vi "PDExitByError.vi"(1 "ExitLimit":dbl, 2 "Time(s)":dbl, 3 "NewValue":dbl) -> (0 "ShouldExit?":bool)   [LabVIEW 2016]
uses:
  <vilib>/Analysis/NI_AALBase.lvlib
  <vilib>/Analysis/baseanly.llb/Mean (DBL).vi
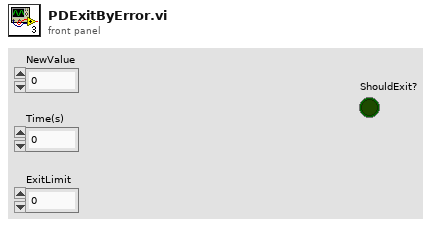
[diagram p1: front panel]
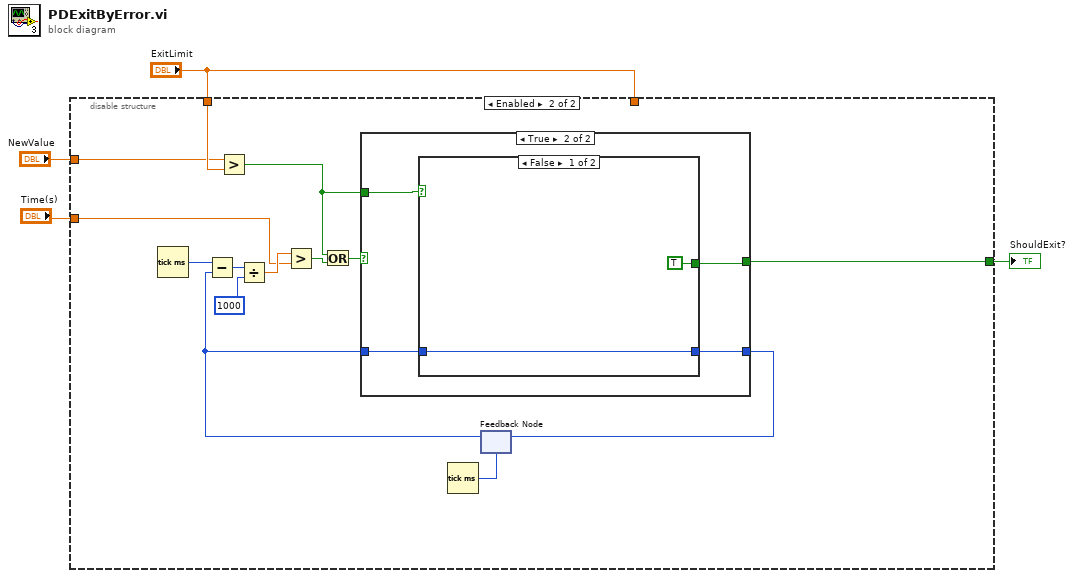
[diagram p0: block diagram]
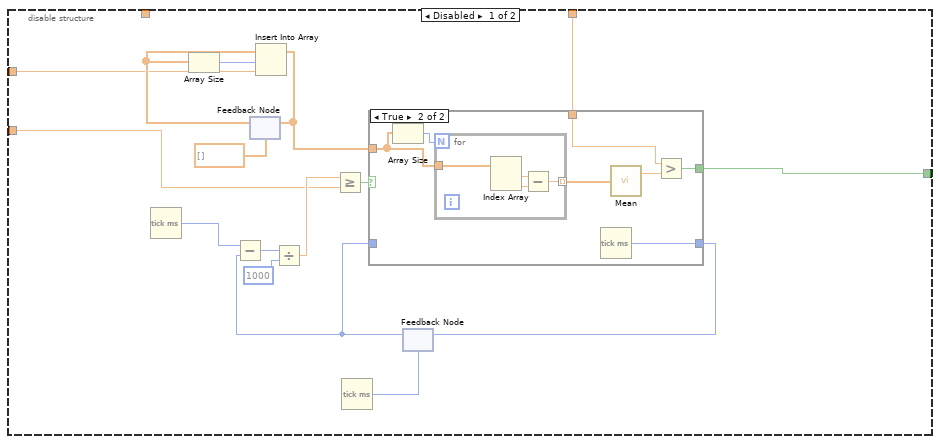
[diagram p2: hidden frame]
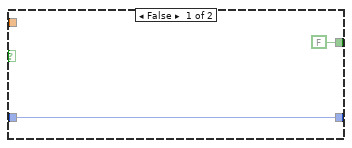
[diagram p3: hidden frame]
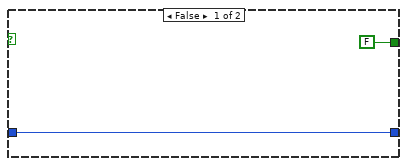
[diagram p4: hidden frame]
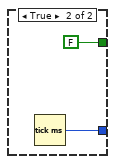
[diagram p5: hidden frame]
diagram:
  n1 = disable-structure shown="Enabled" {
    disable-tunnel: "NewValue" -> [w8 w36]
    disable-tunnel: "Time(s)" -> [w7 w40]
    disable-tunnel: "ExitLimit" -> [w6 _]
    disable-tunnel: "ExitLimit" -> [_ w37]
    disable-tunnel: [w5 w34] -> w1
    frame Disabled {
      n2 = Tick Count (ms)() -> (millisecond timer value=w17:u32)
      n3 = feedback #1(dbl[] []) -> (w10:dbl[])
      n4 = Array Size(array=w10) -> (size(s)=w9:i32)
      n5 = Insert Into Array(array=w10, index=w9, new element=w8) -> (w18:dbl[])
      n6 = feedback-in #1(w18) -> ()
      n7 = Tick Count (ms)() -> (millisecond timer value=w13:u32)
      n8 = feedback #2(w13) -> (w11:u32)
      n9 = Subtract(x=w17, y=w11) -> (x-y=w16:u32)
      n10 = Divide(x=w16, y=u32 1000) -> (x/y=w14:dbl)
      n11 = Greater Or Equal?(x=w14, y=w7) -> (x >= y?=w19:bool)
      n12 = case shown="True" w19 {
        tunnel: w18 -> [_ w25]
        tunnel: [FALSE w27] -> w5
        tunnel: [w21 w24] -> w12
        tunnel: w11 -> [w21 _]
        tunnel: w6 -> [_ w23]
        frame False {
        }
        frame True {
          n13 = Array Size(array=w25) -> (size(s)=w26:i32)
          n14 = for {
            N: w26 -> [_]
            tunnel: w25 -> [w33]
            tunnel: [w30] -> w29 mode=indexing
            n15 = Index Array(array=w33) -> (element #1=w31:dbl, element #2=w32:dbl)  [unwired: 2 in]
            n16 = Subtract(x=w31, y=w32) -> (x-y=w30:dbl)
          }
          n17 = Tick Count (ms)() -> (millisecond timer value=w24:u32)
          n18 = call-poly <vilib>:"Mean.vi"("X"=w29) -> ("mean"=w28:dbl)  [unwired: 1 out]
          n19 = Greater?(x=w23, y=w28) -> (0:w27:bool)
        }
      }
      n20 = feedback-in #2(w12) -> ()
    }
    frame Enabled {
      n21 = Tick Count (ms)() -> (millisecond timer value=w44:u32)
      n22 = Greater?(x=w36, y=w37) -> (0:w35:bool)
      n23 = Tick Count (ms)() -> (millisecond timer value=w47:u32)
      n24 = feedback #3(w47) -> (w45:u32)
      n25 = Subtract(x=w44, y=w45) -> (x-y=w43:u32)
      n26 = Divide(x=w43, y=u32 1000) -> (x/y=w41:dbl)
      n27 = Greater?(x=w41, y=w40) -> (0:w38:bool)
      n28 = Or(x=w35, y=w38) -> (x .or. y?=w39:bool)
      n29 = case shown="True" w39 {
        tunnel: [w49 w53] -> w46
        tunnel: w45 -> [w49 w50]
        tunnel: w35 -> [_ w52]
        tunnel: [FALSE w51] -> w34
        frame False {
        }
        frame True {
          n30 = case shown="False" w52 {
            tunnel: [w54 w57] -> w53
            tunnel: [TRUE FALSE] -> w51
            tunnel: w50 -> [w54 _]
            frame False {
            }
            frame True {
              n31 = Tick Count (ms)() -> (millisecond timer value=w57:u32)
            }
          }
        }
      }
      n32 = feedback-in #3(w46) -> ()
    }
  }
  "ShouldExit?" <- w1
